vi "WriteDigitalOutput.vi"(8 "error in (no error)":errorcluster, 9 "Tristate":bool, 10 "data":bool, 11 "TesteractHAL_DigitalIO In":refnum<class "TesteractHAL_DigitalOutput_EthernetModbus.lvclass">) -> (0 "error out":errorcluster, 3 "TesteractHAL_DigitalIO Out":refnum<class "TesteractHAL_DigitalOutput_EthernetModbus.lvclass">)   [LabVIEW 2017, in "TesteractHAL_DigitalOutput_EthernetModbus.lvlib" / "TesteractHAL_DigitalOutput_EthernetModbus.lvclass"]
doc: "Write a single digital signal."
uses:
  TesteractHAL_DigitalOutput_EthernetModbus.lvclass
  C:/Program Files (x86)/Testeract/HWLib/HAL/Device/TesteractHAL_Device.lvlibp/TesteractHAL_Device.lvclass
  TesteractHAL_DigitalOutput_EthernetModbus.lvclass/TesteractHAL_DigitalOutput_EthernetModbus.ctl
  Program Files (x86)/Testeract/HWLib/HAL/Device/TesteractHAL_Device.lvlibp/ReadConnectionAlias.vi
  Drivers/NIModbus/NI Modbus.llb/MB Ethernet Master Query Write Single Coil (poly).vi
  Program Files (x86)/Testeract/TCPConnectionManager/Testeract_TCPConnectionManager.lvlibp/Testeract_TCPConnectionManager.lvclass
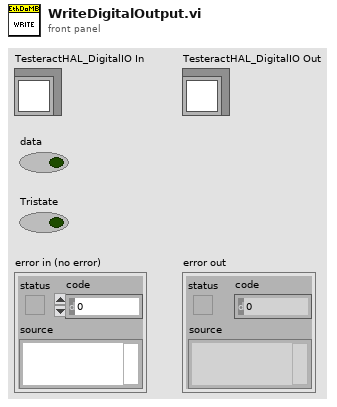
[diagram p1: front panel]
types:
  T1 = typedef "Testeract_TCPConnectionManager.lvlibp/Semaphore RefNum" = refnum<k1>
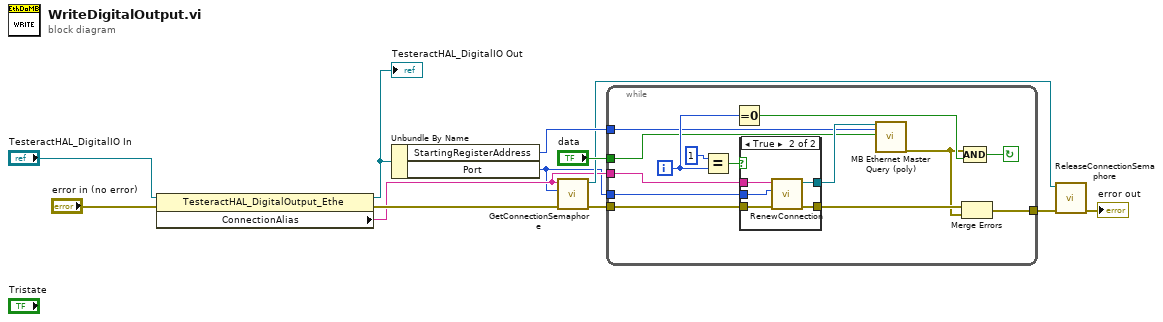
[diagram p0: block diagram]
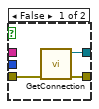
[diagram p2: hidden frame]
diagram:
  n1 = property class="TesteractHAL_DigitalOutput_Ethe"(reference="TesteractHAL_DigitalIO In", error in="error in (no error)") -> (reference out=w11:refnum<class "TesteractHAL_DigitalOutput_EthernetModbus.lvclass">, error out=w5:errorcluster, "ConnectionAlias"=w2:string)
  "TesteractHAL_DigitalIO Out" <- w11
  n2 = Unbundle By Name(w11) -> ("StartingRegisterAddress"=w12:u16, "Port"=w1:u16)
  n3 = call "GetConnectionSemaphore.vi"("error in (no error)"=w5, "Port"=w1, "IPAddress"=w2) -> ("error out"=w4:errorcluster, "Semaphore Ref"=w3:T1)  [unwired: 7 in]
  n4 = while {
    tunnel: w2 -> [w26]
    tunnel: w4 -> [w25]
    tunnel: [w18] -> w7
    tunnel: w12 -> [w15]
    tunnel: w1 -> [w14]
    tunnel: "data" -> [w13]
    i -> [w20]
    stop <- w21 continue-if-true
    n5 = Equal?(x=1, y=w20) -> (x = y?=w23:bool)
    n6 = Equal To 0?(x=w20) -> (x = 0?=w19:bool)
    n7 = case shown="True" w23 {
      tunnel: w26 -> [_ w31]
      tunnel: w25 -> [w29 w34]
      tunnel: [w27 w32] -> w16
      tunnel: [w28 w33] -> w22
      tunnel: w14 -> [_ w30]
      frame False {
        n8 = call "GetConnection.vi"("error in (no error)"=w29) -> ("error out"=w28:errorcluster, "Connection ID"=w27:refnum<k5>)  [unwired: 9 in]
      }
      frame True {
        n9 = call "RenewConnection.vi"("error in (no error)"=w34, "Port"=w30, "IPAddress"=w31) -> ("error out"=w33:errorcluster, "Connection ID"=w32:refnum<k5>)  [unwired: 7 in]
      }
    }
    n10 = call-poly "MB Ethernet Master Query (poly).vi"("TCP Connection Refnum in"=w16, "Address"=w15, "Coil"=w13) -> ("error out"=w17:errorcluster)  [unwired: 2 in, 14 out]
    n11 = Merge Errors(w22, w17) -> (w18:errorcluster)
    n12 = Compound Arithmetic op=AND(w17, w19) -> (w21:bool)
  }
  n13 = call "ReleaseConnectionSemaphore.vi"("error in (no error)"=w7, "Semaphore Refnum"=w3) -> ("error out"=→"error out":errorcluster)  [unwired: 9 in]
